vi "ICMP-Parse.vi"(9 "IPv4 Payload":u8[](array[numeric])=[8, 0, 77, 70, 0, 1, 0, 21, 97, 98, 99, 100, 101, 102, 103, 104, 105, 106, 107, 108, 109, 110, 111, 112, 113, 114, 115, 116, 117, 118, 119, 97, 98, 99, 100, 101, 102, 103, 104, 105] format="%02x") -> (1 "Data":u8[](array[numeric])=[97, 98, 99, 100, 101, 102, 103, 104, 105, 106, 107, 108, 109, 110, 111, 112, 113, 114, 115, 116, 117, 118, 119, 97, 98, 99, 100, 101, 102, 103, 104, 105] format="%02x", 2 "Checksum OK?":bool, 3 "Header":T1={"Type of Message"=8, "Code"=0, "Checksum"=19782, "Quench"=65557} {"Checksum" format="%04x"})   [LabVIEW 2017]
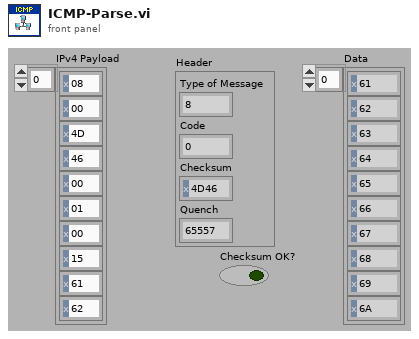
[diagram p1: front panel]
types:
  T1 = cluster{"Type of Message":u8, "Code":u8, "Checksum":u16, "Quench":u32}
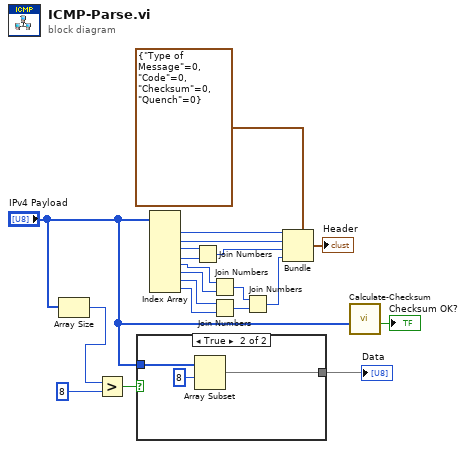
[diagram p0: block diagram]
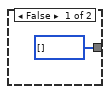
[diagram p2: hidden frame]
diagram:
  n1 = Array Size(array="IPv4 Payload") -> (size(s)=w4:i32)
  n2 = Greater?(x=w4, y=8 ("index")) -> (0:w6:bool)
  n3 = case shown="True" w6 {
    tunnel: "IPv4 Payload" -> [_ w23]
    tunnel: [u8[] [] w22] -> w5
    frame False {
    }
    frame True {
      n4 = Array Subset(array=w23, index=8) -> (w22:u8[])  [unwired: 1 in]
    }
  }
  "Data" <- w5
  n5 = Index Array(array="IPv4 Payload") -> (element #1=w20:u8, element #2=w19:u8, element #3=w17:u8, element #4=w16:u8, element #5=w14:u8, element #6=w13:u8, element #7=w12:u8, element #8=w11:u8)  [unwired: 8 in]
  n6 = Join Numbers(hi=w17, lo=w16) -> ((hi.lo)=w15:u16)
  n7 = Join Numbers(hi=w14, lo=w13) -> ((hi.lo)=w9:u16)
  n8 = Join Numbers(hi=w12, lo=w11) -> ((hi.lo)=w10:u16)
  n9 = Join Numbers(hi=w9, lo=w10) -> ((hi.lo)=w8:u32)
  n10 = Bundle(cluster=T1 {"Type of Message"=0, "Code"=0, "Checksum"=0, "Quench"=0}, "Type of Message"=w20, "Code"=w19, "Checksum"=w15, "Quench"=w8) -> (→"Header":T1)
  n11 = call "Calculate-Checksum.vi"("Array"="IPv4 Payload") -> ("Checksum OK?"=→"Checksum OK?":bool)  [unwired: 9 in, 1 out]
